vi "GetLeCroy_SynthFocus_25_GPU.vi"(1 "Digitizer Settings":T8={"Digitizer delay (us) "=0.0, "rf points per line"=2048, "lines per plane"=128, "Samp Rate (Hz)"=100000000.0, "Additional dig delay (us)"=0.0, "Voltage Scale"=0.4, "Pre-Looks"=0, "Offset delay (us)"=0.0, "bits A/D"=8, "Avg Num"=1, "DigTimeOut"=5.0, "Rel Dig Delay"=0.0, "Dig Ch"=0, "LeCroyCluster"={"LeCroy Channels"=[TRUE, FALSE, FALSE, FALSE], "LC read pt offset"=0.0, "Sweep Avg"=FALSE}, "Main Digitizer"=enum."NI Digitizer", "Dig Config"=enum."Single channel", "Digitizer ID Cluster"={"Acqiris/Alazar/SP ID"=[], "NI Instr Handles"=[], "LeCroy VISA"="", "GaGe Handle"={"Handle"=0, "Sample size"=0, "Resolution"=0, "Offset"=0, "Channels"=0, "Boards"=0}, "ATS Ref"="ATS9350", "Acqiris Address"=["PCI::INSTR0"], "ADQRef"=refnum, "adq_cu_ptr"=refnum}, "Trigger Settings"={"Trig Source"=1, "Trig Coupling"=0, "Trig Slope"=0, "Level (mV)"=1500.0}, "Bulk Acq"=FALSE, "Bulk Start Indexes"=[], "Data Ref RF"=refnum, "NI ID/Channel"=[], "Total Dig CH"=1, "Xtra Ann Trig delay (us)"=10.0, "Fix Z Delay?"=FALSE, "One Way Transmission?"=FALSE, "Data Ref Log"=refnum} {"Trigger Settings"."Trig Slope" items=["Positive", "Negative"]; "Trigger Settings"."Level (mV)" format="%.2f"; "Trigger Settings"."Trig Coupling" items=["DC 1 MOhm", "AC 1 MOhm", "DC 50 Ohm", "AC 50 Ohm"]; "Trigger Settings"."Trig Source" items=["Chan 1", "External"]; "Rel Dig Delay" format="%.2f"; "DigTimeOut" format="%.2f"; "Avg Num" min=1; "Offset delay (us)" format="%.2f"; "Additional dig delay (us)" format="%.2f"; "Digitizer delay (us)" format="%.2f"}, 5 "errorin":errorcluster, 7 "Ann Array Params":T5={"Synth Foc?"=FALSE, "Focal Zones"=41, "Switch T/R"=0, "Trans Geometry (mm)"={"Transducer"=0, "Geo Focus"=12.0, "a (radius)"=3.0, "# of rings"=5, "kerf space "=0.1, "Center Freq"=12.0}, "Sub Ap Excite?"=FALSE, "Full Array Scan?"=FALSE, "Xmt/Rcv"={"XMIT"=[TRUE, TRUE, TRUE, TRUE, TRUE], "RCV"=[TRUE, TRUE, TRUE, TRUE, TRUE]}, "PulseSpacing (us)"=0.0, "Xmit Ring"=0, "XMIT CHS"=0, "RCV CHS"=0, "GPU?"=FALSE, "Save TIFF?"=FALSE, "downfactor"=1, "RCV 1CH"=0} {"RCV 1CH" items=["All", "1", "2", "3", "4", "5"]; "Trans Geometry (mm)"."Transducer" items=["6D 12R 40 MHz"=0, "10D 31R 20 MHz"=1, "10D 23R 20 MHz"=2, "6D 23R 40 MHz"=3, "4.5D 10.7R 40 MHz"=4, "9D 23.5R 20 MHz"=5, "9D 25.8R 20MHz"=6, "Enter"=99]; "Switch T/R" min=1 max=5 step=1}, 11 "Reverse?":bool) -> (12 "Gain Array":T12(array[cluster]), 13 "Raw VGain (scale)":dbl, 15 "VGain (dB)":dbl, 19 "error out":errorcluster)   [LabVIEW 2022 SP3]
uses:
  -DigitizerRoutines/DigitizerSettings.ctl
  -DigitizerRoutines/Digitizer.ctl
  -DigitizerRoutines/DigConfig.ctl
  -DigitizerRoutines/DigitizerID.ctl
  C:/Windows/System32/ADQAPI_dotNet_helper.dll
  Windows/System32/ADQAPI_dotNet_helper.dll
  Annular Array/-AnnularRoutines/AnnularArray.ctl
  Annular Array/-AnnularRoutines/TransGeometry.ctl
  Annular Array/-AnnularRoutines/ArrayGeometry.ctl
  Motion Controllers/NI_controller/-NI_MotionRoutines/MotionParameters.ctl
  Motion Controllers/NI_controller/-NI_MotionRoutines/MotionSys.ctl
  Motion Controllers/-MotionRoutines/ScanAxis.ctl
  Motion Controllers/-MotionRoutines/3rdAxis.ctl
panel:
  in  "Motion Settings":T1={"No Motion?"=FALSE, "Motion System"=enum."NI 735x", "Motion Bd ID"=1, "Motion Profile"="SMAC1", "# Axis"=1, "Reverse Z axis?"=TRUE, "SMAC Axis"=0, "scan pair"=enum."y-(x) scan", "RT fps"=6.0, "Steps per mm"=[1000, 1000, 1000, 1000], "Motor Parameters"={"velocity ct/s"=[10000.0, 10000.0, 10000.0, 50000.0], "accel ct/s^2"=[50000.0, 50000.0, 50000.0, 200000.0]}, "One Way Scan"=FALSE, "Reverse One Way Scan"=FALSE, "Global Position (mm)"=[], "Plane"=0, "Distance between\nscan lines (um)"=0.0, "Distance between\nscan planes (um)"=0.0, "number of scan planes"=1, "Total steps in line"=0, "Xtra plane\ndistance  (um)"=100, "Xtra planes "=1, "Add Axis"=FALSE, "overshoot cts"=200, "BKPT Shift"=0, "Scan Start Time (ms)"=0, "ESP VISA"="GPIB::1::INSTR", "3rd Axis"=1, "GL Ref Out"=refnum, "Galil Address"=""} {"3rd Axis" items=["x", "y", "z", "w"]; "Xtra planes" min=1; "Xtra plane\ndistance  (um)" min=0; "Distance between\nscan planes (um)" format="%.2f"; "Distance between\nscan lines (um)" format="%.2f"; "SMAC Axis" items=["None"=0, "Axis 1"=1, "Axis 2"=2, "Axis 3"=3, "Axis 4"=4, "Axis 5"=5, "Axis 6"=6, "Axis 7"=7, "Axis 8"=8, "Vector Space 1"=17, "Vector Space 2"=18, "Vector Space 3"=19, "Vector Space 4"=20]; "Motion Bd ID" min=1 max=32 step=1}
  out "Synth focus time time":u32
  # "1-D and 2-D B scan settings"
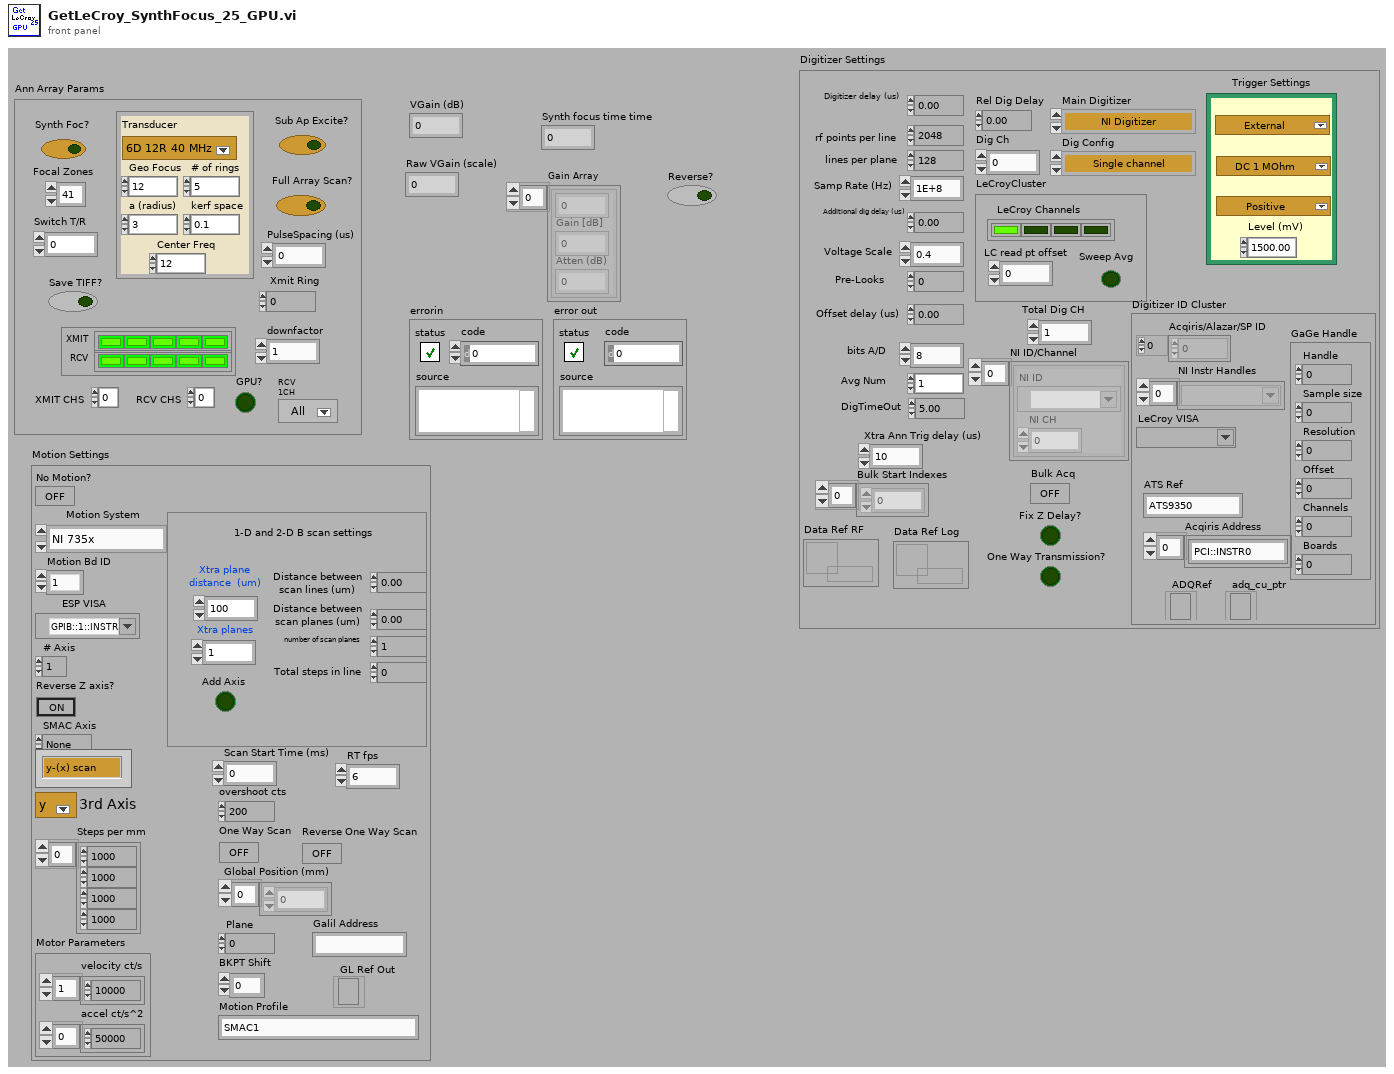
[diagram p1: front panel]
types:
  T1 = typedef "MotionParameters.ctl" = cluster{"No Motion?":bool, "Motion System":T2, "Motion Bd ID":u8, "Motion Profile":string, "# Axis":i8, "Reverse Z axis?":bool, "SMAC Axis":u16, "scan pair":T3, "RT fps":sgl, "Steps per mm":i32[], "Motor Parameters":cluster{"velocity ct/s":dbl[], "accel ct/s^2":dbl[]}, "One Way Scan":bool, "Reverse One Way Scan":bool, "Global Position (mm)":dbl[], "Plane":i32, "Distance between\nscan lines (um)":sgl, "Distance between\nscan planes (um)":sgl, "number of scan planes":i32, "Total steps in line":i32, "Xtra plane\ndistance  (um)":i32, "Xtra planes ":i32, "Add Axis":bool, "overshoot cts":i32, "BKPT Shift":i32, "Scan Start Time (ms)":u32, "ESP VISA":refnum<visa-resource-name>, "3rd Axis":T4, "GL Ref Out":refnum<k7>, "Galil Address":string}
  T2 = typedef "MotionSys.ctl" = enum16{"MM3000", "NI 735x", "Newport ESP", "No Motion Card", "Galil"}
  T3 = typedef "ScanAxis.ctl" = enum16{"y-(x) scan", "x-(y) scan", "z-(x) scan", "z-(y) scan", "y-(z) scan", "x-(z) scan", "w-(x) scan", "w-(y) scan", "w-(z) scan", "x-(w) scan", "y-(w) scan", "z-(w) scan"}
  T4 = typedef "3rdAxis.ctl" = u16
  T5 = typedef "AnnularArray.ctl" = cluster{"Synth Foc?":bool, "Focal Zones":i16, "Switch T/R":i16, "Trans Geometry (mm)":T6, "Sub Ap Excite?":bool, "Full Array Scan?":bool, "Xmt/Rcv":cluster{"XMIT":bool[], "RCV":bool[]}, "PulseSpacing (us)":sgl, "Xmit Ring":i32, "XMIT CHS":u8, "RCV CHS":u8, "GPU?":bool, "Save TIFF?":bool, "downfactor":i32, "RCV 1CH":u16}
  T6 = typedef "TransGeometry.ctl" = cluster{"Transducer":T7, "Geo Focus":dbl, "a (radius)":dbl, "# of rings":i32, "kerf space ":dbl, "Center Freq":dbl}
  T7 = typedef "ArrayGeometry.ctl" = u16
  T8 = typedef "DigitizerSettings.ctl" = cluster{"Digitizer delay (us) ":dbl, "rf points per line":i32, "lines per plane":i32, "Samp Rate (Hz)":dbl, "Additional dig delay (us)":dbl, "Voltage Scale":dbl, "Pre-Looks":i32, "Offset delay (us)":dbl, "bits A/D":i8, "Avg Num":i32, "DigTimeOut":sgl, "Rel Dig Delay":sgl, "Dig Ch":i32, "LeCroyCluster":cluster{"LeCroy Channels":bool[], "LC read pt offset":dbl, "Sweep Avg":bool}, "Main Digitizer":T9, "Dig Config":T10, "Digitizer ID Cluster":T11, "Trigger Settings":cluster{"Trig Source":u16, "Trig Coupling":u16, "Trig Slope":u16, "Level (mV)":dbl}, "Bulk Acq":bool, "Bulk Start Indexes":i32[], "Data Ref RF":refnum<data-value>, "NI ID/Channel":cluster{"NI ID":refnum<k15>, "NI CH":i32}[], "Total Dig CH":i32, "Xtra Ann Trig delay (us)":dbl, "Fix Z Delay?":bool, "One Way Transmission?":bool, "Data Ref Log":refnum<data-value>}
  T9 = typedef "Digitizer.ctl" = enum16{"Acqiris Digitizer", "NI Digitizer", "LeCroy", "GaGe", "AlazarTech", "No Digitizer", "Teledyne"}
  T10 = typedef "DigConfig.ctl" = enum16{"Single channel", "2 Chans w/ 2 Acqiris", "2 Chans w/ 1 Acqiris", "5-CH Pulser New", "5-CH pulser w/ ann array", "5-pass style ann array", "Empty"}
  T11 = typedef "DigitizerID.ctl" = cluster{"Acqiris/Alazar/SP ID":u32[], "NI Instr Handles":refnum<k15>[], "LeCroy VISA":refnum<visa-resource-name>, "GaGe Handle":cluster{"Handle":u32, "Sample size":u32, "Resolution":i32, "Offset":i32, "Channels":u32, "Boards":u32}, "ATS Ref":string, "Acqiris Address":string[], "ADQRef":refnum<k24>, "adq_cu_ptr":refnum<k24>}
  T12 = cluster{sgl, "Gain [dB]  ":sgl, "Atten (dB)":sgl}[]
  T13 = cluster{sgl, "Gain [dB]  ":sgl, "Atten (dB)":sgl}
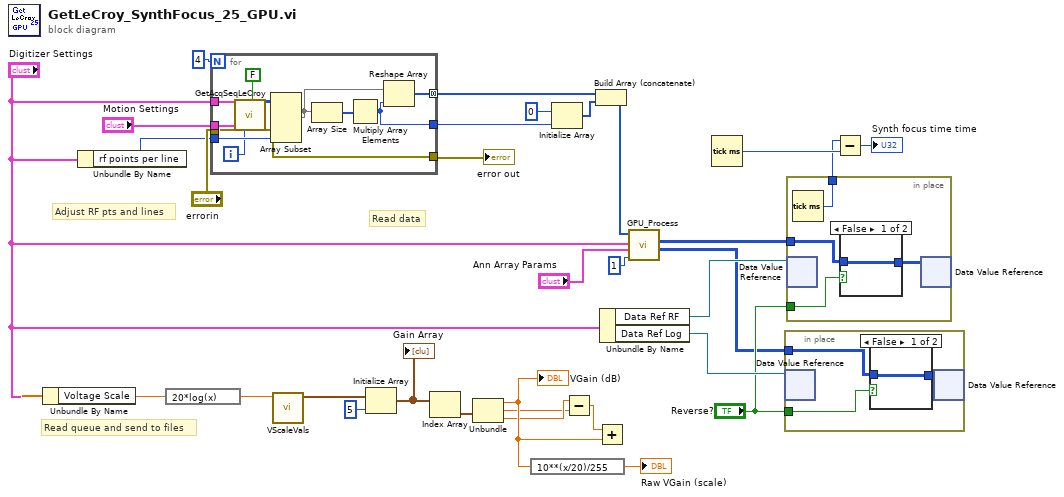
[diagram p0: block diagram]
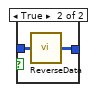
[diagram p2: hidden frame]
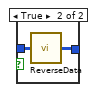
[diagram p3: hidden frame]
diagram:
  # "Read data"
  # "Adjust RF pts and lines"
  # "Read queue and send to files"
  n1 = Unbundle By Name("Digitizer Settings") -> ("Voltage Scale"=w23:dbl)
  n2 = Unbundle By Name("Digitizer Settings") -> ("rf points per line"=w7:i32)
  n3 = expression code="20*log(x)"(w23) -> (w24:dbl)
  n4 = for {
    N: 4 -> [_]
    tunnel: "errorin" -> [w43]
    tunnel: "Motion Settings" -> [w42]
    tunnel: "Digitizer Settings" -> [w41]
    tunnel: w7 -> [w39]
    tunnel: [w38] -> w6
    tunnel: [w35] -> w2
    tunnel: [w34] -> w1 mode=concatenating
    i -> [w33]
    n5 = call "GetAcqSeqLeCroy.vi"("Digitizer Settings"=w41, "Motion Settings"=w42, "errorin"=w43, "Source (0: Channel 1)"=w33, "save?"=FALSE) -> ("Data Array"=w40:i16[][], "error out"=w38:errorcluster)  [unwired: 16 in, 5 out]
    n6 = Array Subset(array=w40, length (col)=w39) -> (w36:i16[][])  [unwired: 3 in]
    n7 = Array Size(array=w36) -> (size(s)=w37:i32[])
    n8 = Multiply Array Elements(1:w37) -> (0:w35:i32)
    n9 = Reshape Array(w36, w35) -> (w34:i16[])
  }
  "error out" <- w6
  n10 = call "VScaleVals.vi"("Full Scale"=w24) -> ("Voltage Scale"=w17:T13)  [unwired: 8 in, 2 out]
  n11 = Initialize Array(w17, 5 ("dimension size")) -> (w15:T12)
  "Gain Array" <- w15
  n12 = Index Array(array=w15) -> (element=w32:T13)  [unwired: 1 in]
  n13 = Unbundle(w32) -> (w31:sgl, "Gain [dB]"=w29:sgl, "Atten (dB)"=w30:sgl)
  "VGain (dB)" <- w31
  n14 = expression code="10**(x/20)/255"(w31) -> (→"Raw VGain (scale)":sgl)
  n15 = Initialize Array(i16 0 ("Numeric"), w2) -> (w5:i16[])
  n16 = Subtract(x=w30, y=w29) -> (x-y=w28:sgl)
  n17 = Build Array (concatenate)(w1, w5) -> (w4:i16[])
  n18 = Add(x=w28, y=w31) -> ()  [unwired: 1 out]
  n19 = Unbundle By Name("Digitizer Settings") -> ("Data Ref RF"=w21:refnum<data-value>, "Data Ref Log"=w20:refnum<data-value>)
  n20 = call "GPU_Process.vi"("DataFlag"=1, "Ann Array Params"="Ann Array Params", "Digitizer Settings"="Digitizer Settings", "Raw Data In"=w4) -> ("RFimageData"=w13:i16[][], "RF_Out"=w14:i16[][])  [unwired: 5 in, 1 out]
  n21 = Tick Count (ms)() -> (millisecond timer value=w26:u32)
  n22 = in-place {
    in-place-border: w13 -> [w46]
    in-place-border: "Reverse?" -> [w45]
    n23 = in-place-dvr #1(w20) -> ()  [unwired: 2 out]
    n24 = case shown="False" w45 {
      tunnel: w46 -> [w48 w50]
      tunnel: [w48 w49] -> w47
      frame False {
      }
      frame True {
        n25 = call "ReverseData.vi"("Array in"=w50) -> ("Array out"=w49:i16[][])
      }
    }
    n26 = in-place-dvr #1(w47) -> ()  [unwired: 2 out]
  }
  n27 = in-place {
    in-place-border: w14 -> [w52]
    in-place-border: [w54] -> w19
    in-place-border: "Reverse?" -> [w51]
    n28 = in-place-dvr #2(w21) -> ()  [unwired: 2 out]
    n29 = Tick Count (ms)() -> (millisecond timer value=w54:u32)
    n30 = case shown="False" w51 {
      tunnel: w52 -> [w55 w57]
      tunnel: [w55 w56] -> w53
      frame False {
      }
      frame True {
        n31 = call "ReverseData.vi"("Array in"=w57) -> ("Array out"=w56:i16[][])
      }
    }
    n32 = in-place-dvr #2(w53) -> ()  [unwired: 2 out]
  }
  n33 = Subtract(x=w19, y=w26) -> (x-y=→"Synth focus time time":u32)
